vi "AddLibSectionIfMissing.vi"(8 "error in (no error)":errorcluster, 10 "LibraryName":string="ModuleA", 11 "Config Refnum in":T1) -> (0 "error out":errorcluster, 3 "Config Refnum out":T1)   [LabVIEW 2023, in "Reusables.lvlib"]
uses:
  Reusables.lvlib
  <vilib>/Utility/config.llb/Config Data RefNum.ctl
  <vilib>/Utility/config.llb/Write Key (String).vi
  <vilib>/Utility/config.llb/NI_LVConfig.lvlib
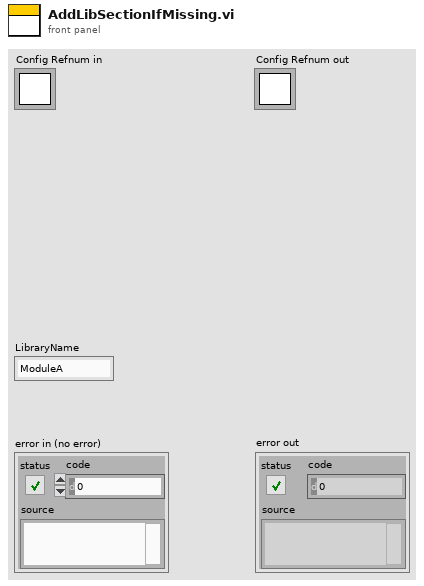
[diagram p1: front panel]
types:
  T1 = typedef "NI_LVConfig.lvlib/Config Data RefNum.ctl" = refnum<k1>
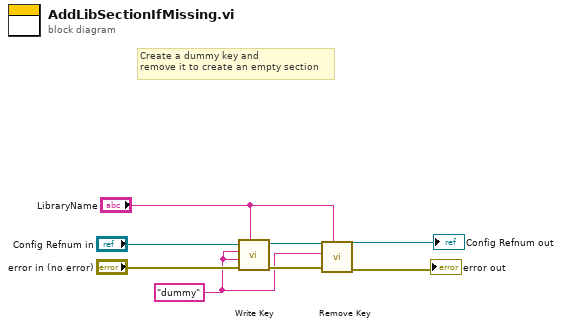
[diagram p0: block diagram]
diagram:
  w4 = "dummy" ("key")
  # "Create a dummy key and\nremove it to create an empty section"
  n1 = call-poly <vilib>:"Write Key.vi"("section"="LibraryName", "error in (no error)"="error in (no error)", "value"=w4, "key"=w4, "refnum"="Config Refnum in") -> ("error out"=w5:errorcluster, "refnum out"=w6:T1)  [unwired: 4 in, 1 out]
  n2 = call <vilib>:"Remove Key.vi"("section"="LibraryName", "error in (no error)"=w5, "key"=w4, "refnum"=w6) -> ("error out"=→"error out":errorcluster, "refnum out"=→"Config Refnum out":T1)  [unwired: 5 in, 1 out]
